vi "GetLockedStatus.vi"(0 "Filename":string) -> (1 "Locked?":bool, 2 "locked name":string, 3 "Cleaned":string)   [LabVIEW 2012]
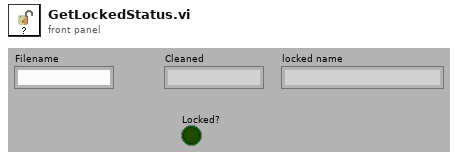
[diagram p1: front panel]
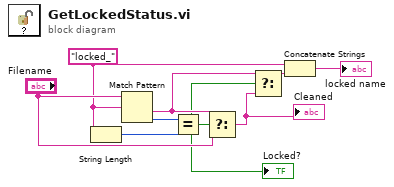
[diagram p0: block diagram]
diagram:
  w5 = "locked_" ("regular expression")
  n1 = String Length(string=w5) -> (length=w4:i32)
  n2 = Match Pattern(string="Filename", regular expression=w5) -> (after substring=w7:string, offset past match=w6:i32)  [unwired: 1 in, 2 out]
  n3 = Equal?(x=w6, y=w4) -> (x = y?=w3:bool)
  "Locked?" <- w3
  n4 = Select(t=w7, s=w3, f="Filename") -> (s? t:f=w1:string)
  "Cleaned" <- w1
  n5 = Select(t=w7, s=w3, f=w1) -> (s? t:f=w9:string)
  n6 = Concatenate Strings(w5, w9) -> (→"locked name":string)
